vi "get_libraryWhitelist.vi"(0 "Host_Reference":refnum<class "HGF_Reference.lvclass">, 2 "timeout in ms (-1)":i32=-1, 5 "error in (no error)":errorcluster) -> (14 "dup Host_Reference":refnum<class "HGF_Reference.lvclass">, 16 "Library Whitelist":string[](array[string]), 19 "error out":errorcluster)   [LabVIEW 2009, in "MoAgSy.lvlib" / "MoAgSy_Host.lvclass"]
doc: "<B>public</B> VI returns referenced Hosts whitelisted libraries.\nAgents that belong to whitelisted libraries will be startet at this host irrespective of the hosts security settings.\n\nF.Berck@gsi.de\nGSI Darmstadt 2009"
uses:
  MoAgSy_Host.lvclass
  HGF_BaseClasses/HGF_Reference/HGF_Reference.lvclass
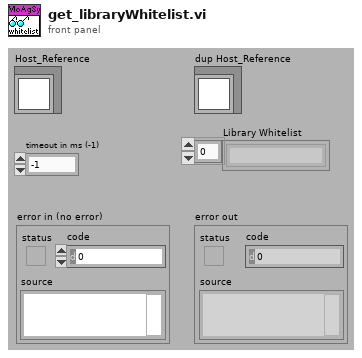
[diagram p1: front panel]
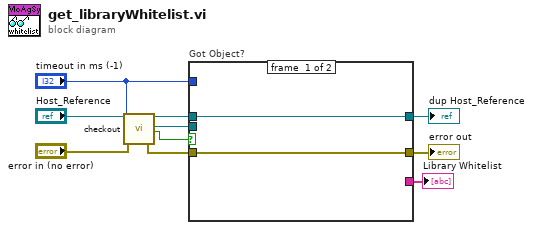
[diagram p0: block diagram]
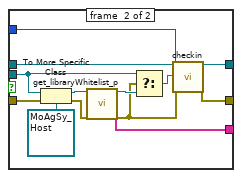
[diagram p2: hidden frame]
diagram:
  n1 = call "checkout.vi"("HGF_Reference"="Host_Reference", "timeout in ms (-1)"="timeout in ms (-1)", "error in (no error)"="error in (no error)") -> ("dup HGF_Reference"=w7:refnum<class "HGF_Reference.lvclass">, "Object"=w4:refnum<class>, "got object?"=w6:bool, "error out"=w3:errorcluster)  [unwired: 13 out]
  n2 = case "Got Object?" shown="True" w6 {
    tunnel: w3 -> [w11 w25]
    tunnel: w4 -> [_ w19]
    tunnel: w7 -> [w12 w23]
    tunnel: [w12 w22] -> w8
    tunnel: "timeout in ms (-1)" -> [_ w21]
    tunnel: [w11 w20] -> w10
    tunnel: [_ w14] -> w1
    frame #0 {
    }
    frame #1 {
      n3 = To More Specific Class(target class=refnum<class "MoAgSy_Host.lvclass"> refnum ("MoAgSy.lvlib:MoAgSy_Host.lvclass"), reference=w19, error in=w25) -> (specific class reference=w17:refnum<class "MoAgSy_Host.lvclass">, error out=w13:errorcluster)
      n4 = call "get_libraryWhitelist_p.vi"("MoAgSy_Host"=w17, "error in (no error)"=w13) -> ("dup MoAgSy_Host"=w16:refnum<class "MoAgSy_Host.lvclass">, "Library Whitelist"=w14:string[], "error out"=w15:errorcluster)  [unwired: 15 out]
      n5 = Select(t=w19, s=w15, f=w16) -> (s? t:f=w18:refnum<class>)
      n6 = call "checkin.vi"("HGF_Reference"=w23, "Object"=w18, "timeout /ms (-1)"=w21, "error in (no error)"=w15) -> ("dup HGF_Reference"=w22:refnum<class "HGF_Reference.lvclass">, "error out"=w20:errorcluster)  [unwired: 14 out]
    }
  }
  "dup Host_Reference" <- w8
  "error out" <- w10
  "Library Whitelist" <- w1
